vi "Create.vi"(8 "Error In":errorcluster, 10 "ICommunicate":refnum<class "ICommunicate.lvclass">) -> (0 "Error Out":errorcluster, 3 "SDO Manager":refnum<class "SDO Manager.lvclass">)   [LabVIEW 2020, in "CANopen.lvlib" / "SDO Manager.lvlib" / "SDO Manager.lvclass"]
uses:
  SDO Manager.lvclass
  HAL/Source/Interfaces/ICommunicate/ICommunicate.lvclass
  SDO Transfer/SDO Transfer.lvclass
  Response Matcher/Response Matcher.lvclass
  C:/Program Files/National Instruments/LabVIEW 2026/vi.lib/ActorFramework/Actor/Actor.lvclass
  <vilib>/ActorFramework/Message Enqueuer/Message Enqueuer.lvclass
  Response Matcher/Response Matcher.lvclass/Response Matcher.ctl
  SDO Manager.lvclass/SDO Manager.ctl
  HAL/Source/Interfaces/IMessage/IMessage.lvclass
  <vilib>/ActorFramework/Actor/Actor.lvclass
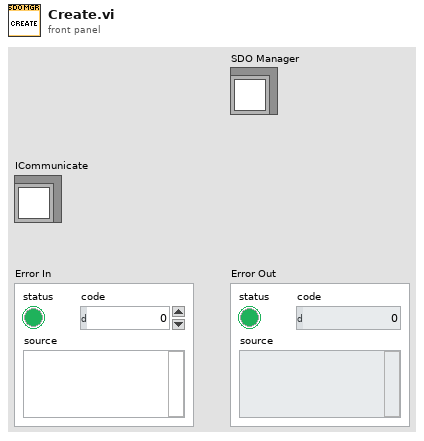
[diagram p1: front panel]
types:
  T1 = map{u8, refnum<class "Message Enqueuer.lvclass">}
  T2 = map{string, refnum<class "SDO Transfer.lvclass">}
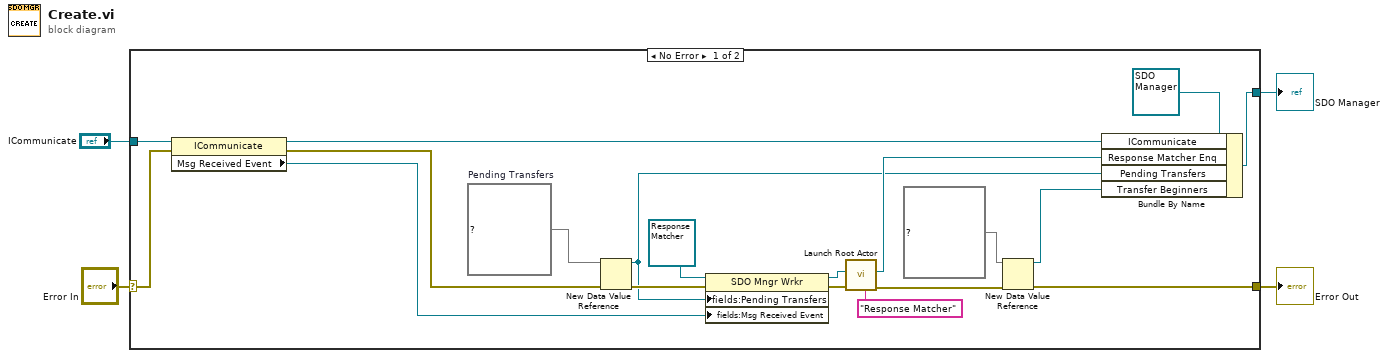
[diagram p0: block diagram]
diagram:
  n1 = case shown="No Error" "Error In" {
    selector: "Error In" -> [w18 w24]
    tunnel: [w6 w24] -> w3
    tunnel: [w17 _] -> w2
    tunnel: "ICommunicate" -> [w11 _]
    frame No Error {
      w23 = T2 {}  # Pending Transfers
      n2 = property class="ICommunicate"(reference=w11, error in=w18) -> (reference out=w10:refnum<class "ICommunicate.lvclass">, error out=w12:errorcluster, "Msg Received Event"=w9:refnum<user-event>)
      n3 = New Data Value Reference(data value=w23, error in=w12) -> (data value reference=w13:refnum<data-value>, error out=w20:errorcluster)
      n4 = property class="SDO Mngr Wrkr"(reference=refnum<class "Response Matcher.lvclass"> refnum ("CANopen Master:SDO Mngr Wrkr"), error in=w20, "fields:Pending Transfers"=w13, "fields:Msg Received Event"=w9) -> (reference out=w14:refnum<class "Response Matcher.lvclass">, error out=w16:errorcluster)
      n5 = call <vilib>:"Launch Root Actor.vi"("Debug Alias"="Response Matcher", "error in (no error)"=w16, "Actor"=w14) -> ("error out"=w7:errorcluster, "Actor's Enqueuer"=w21:refnum<class "Message Enqueuer.lvclass">)  [unwired: 7 in]
      n6 = New Data Value Reference(data value=T1 {} ("Transfer Beginners"), error in=w7) -> (data value reference=w5:refnum<data-value>, error out=w6:errorcluster)
      n7 = Bundle By Name(cluster=refnum<class "SDO Manager.lvclass"> refnum ("reference out"), "ICommunicate"=w10, "Response Matcher Enq"=w21, "Pending Transfers"=w13, "Transfer Beginners"=w5) -> (w17:refnum<class "SDO Manager.lvclass">)
    }
    frame Error {
      # "VI-TechBaseTemplate_Simple_4x4x4"
    }
  }
  "Error Out" <- w3
  "SDO Manager" <- w2
